vi "8channel_ADS_filters.vi"(7 "Apply":bool, 8 "Filters":T2, 10 "Sampling frequency":dbl, 11 "Data in 8 ch":T1) -> (3 "Filtered data array":dbl[](array[numeric]))   [LabVIEW 2023]
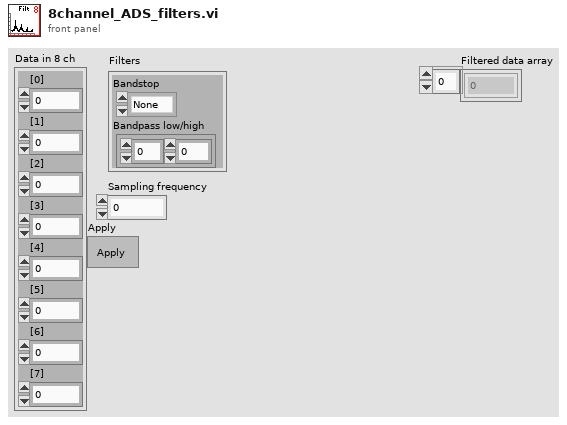
[diagram p1: front panel]
types:
  T1 = cluster{"[0]":dbl, "[1]":dbl, "[2]":dbl, "[3]":dbl, "[4]":dbl, "[5]":dbl, "[6]":dbl, "[7]":dbl}
  T2 = cluster{"Bandstop":enum16{"None", "50", "50 x N"}, "Bandpass low/high":cluster{i32, i32}}
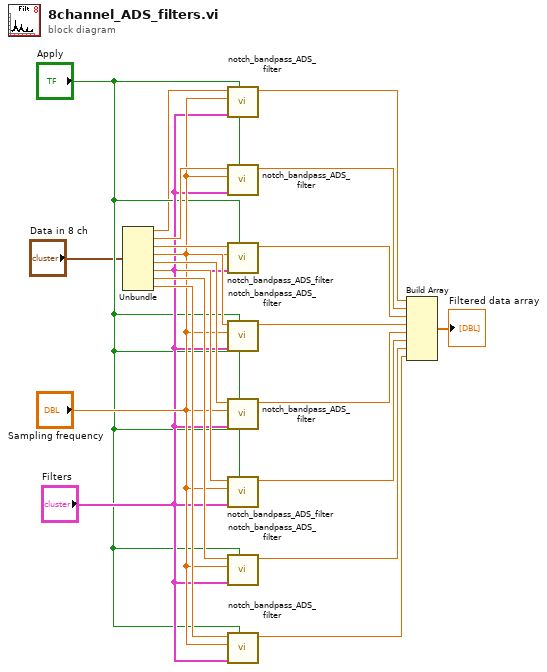
[diagram p0: block diagram]
diagram:
  n1 = Unbundle("Data in 8 ch") -> ("[0]"=w1:dbl, "[1]"=w21:dbl, "[2]"=w20:dbl, "[3]"=w15:dbl, "[4]"=w16:dbl, "[5]"=w17:dbl, "[6]"=w18:dbl, "[7]"=w19:dbl)
  n2 = call "notch_bandpass_ADS_filter.vi"("Apply"="Apply", "Filters"="Filters", "Sampling frequency"="Sampling frequency", "Data in"=w1) -> ("Filtered x"=w14:dbl)  [unwired: 7 in]
  n3 = call "notch_bandpass_ADS_filter.vi"("Apply"="Apply", "Filters"="Filters", "Sampling frequency"="Sampling frequency", "Data in"=w21) -> ("Filtered x"=w13:dbl)  [unwired: 7 in]
  n4 = call "notch_bandpass_ADS_filter.vi"("Apply"="Apply", "Filters"="Filters", "Sampling frequency"="Sampling frequency", "Data in"=w20) -> ("Filtered x"=w12:dbl)  [unwired: 7 in]
  n5 = call "notch_bandpass_ADS_filter.vi"("Apply"="Apply", "Filters"="Filters", "Sampling frequency"="Sampling frequency", "Data in"=w15) -> ("Filtered x"=w11:dbl)  [unwired: 7 in]
  n6 = call "notch_bandpass_ADS_filter.vi"("Apply"="Apply", "Filters"="Filters", "Sampling frequency"="Sampling frequency", "Data in"=w16) -> ("Filtered x"=w10:dbl)  [unwired: 7 in]
  n7 = call "notch_bandpass_ADS_filter.vi"("Apply"="Apply", "Filters"="Filters", "Sampling frequency"="Sampling frequency", "Data in"=w17) -> ("Filtered x"=w9:dbl)  [unwired: 7 in]
  n8 = call "notch_bandpass_ADS_filter.vi"("Apply"="Apply", "Filters"="Filters", "Sampling frequency"="Sampling frequency", "Data in"=w18) -> ("Filtered x"=w8:dbl)  [unwired: 7 in]
  n9 = call "notch_bandpass_ADS_filter.vi"("Apply"="Apply", "Filters"="Filters", "Sampling frequency"="Sampling frequency", "Data in"=w19) -> ("Filtered x"=w7:dbl)  [unwired: 7 in]
  n10 = Build Array(w14, w13, w12, w11, w10, w9, w8, w7) -> (→"Filtered data array":dbl[])
